vi "CameraKill.vi"(8 "error in (no error)":errorcluster, 11 "AndorSDK3 in":refnum<class "Andor3.lvclass">) -> (0 "error out":errorcluster, 3 "AndorSDK3 out":refnum<class "Andor3.lvclass">)   [LabVIEW 2010, in "Andor3.lvclass"]
uses:
  Andor3.lvclass
  Andor3.lvclass/Andor3.ctl
  <userlib>/atcoreA/atcoreA.lvlib
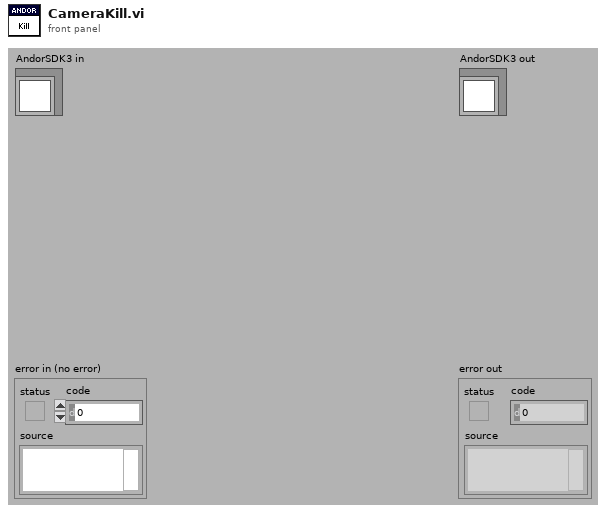
[diagram p1: front panel]
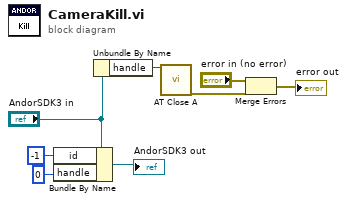
[diagram p0: block diagram]
diagram:
  n1 = Bundle By Name(cluster="AndorSDK3 in", "id"=-1, "handle"=0) -> (→"AndorSDK3 out":refnum<class "Andor3.lvclass">)
  n2 = Unbundle By Name("AndorSDK3 in") -> ("handle"=w8:i32)
  n3 = call <userlib>:"AT Close A.vi"("Hndl"=w8) -> ("error out"=w7:errorcluster)  [unwired: 10 in]
  n4 = Merge Errors("error in (no error)", w7) -> (→"error out":errorcluster)
